vi "Read Z_state.vi"(8 "error in (no error)":errorcluster, 11 "HE_state in":refnum<class "HE_state_v2.lvclass">) -> (0 "error out":errorcluster, 2 "Z_State":T1=enum."on min", 3 "HE_state out":refnum<class "HE_state_v2.lvclass">)   [LabVIEW 2019]
uses:
  Z_state_v2/HE_Z_state_v2.lvclass
  HE_state_v2.lvclass
  C:/my_projects/projects/Algorithms/Labview/19/Heating/heating1/Z_state_v2/HE_Z_state_v2.lvclass
  C:/my_projects/projects/Algorithms/Labview/19/Heating/heating1/ZM_state/HE_ZM_state.lvclass
  C:/my_projects/projects/Algorithms/Labview/19/Sequence/State/State.lvclass
  ctl/Z_State.ctl
  Heating.lvlib
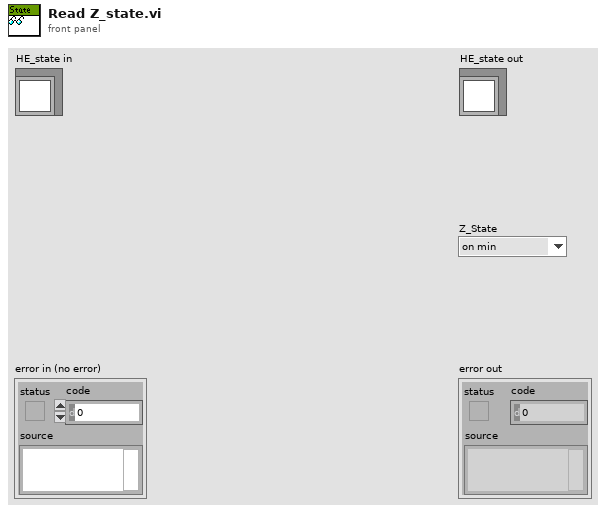
[diagram p1: front panel]
types:
  T1 = typedef "Heating.lvlib/Z_State.ctl" = enum8{"initialization", "alarm", "disabled", "not ready", "stop ready", "reserv", "switched off", "reserv2", "switched on", "check", "on min", "decrease out", "on", "increase out", "on max"}
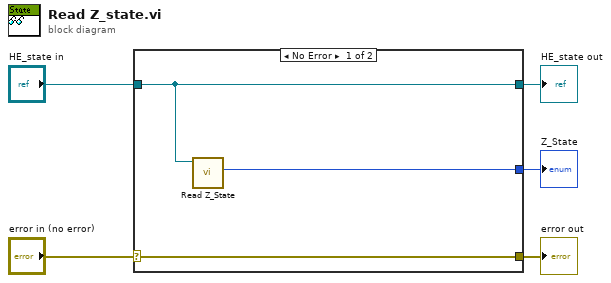
[diagram p0: block diagram]
diagram:
  n1 = case shown="No Error" "error in (no error)" {
    selector: "error in (no error)" -> [w8 w9]
    tunnel: [w8 w9] -> w4
    tunnel: [w6 w10] -> w2
    tunnel: "HE_state in" -> [w6 w10]
    tunnel: [w7 _] -> w1
    frame No Error {
      n2 = call "Read Z_State.vi"("HE1_Z_state in"=w6) -> ("Z_State_heating"=w7:T1)  [unwired: 9 in, 1 out]
    }
    frame Error {
    }
  }
  "error out" <- w4
  "HE_state out" <- w2
  "Z_State" <- w1
